vi "Compile Settings.vi"(8 "error in (no error)":errorcluster, 11 "Plugin in":refnum<class "Output Sequencer.lvclass">) -> (0 "error out":errorcluster, 3 "Plugin out":refnum<class "Output Sequencer.lvclass">)   [LabVIEW 2024, in "Output Sequencer.lvlib" / "Output Sequencer.lvclass"]
uses:
  Output Sequencer.lvclass
  Output Sequencer.lvclass/Output Sequencer.ctl
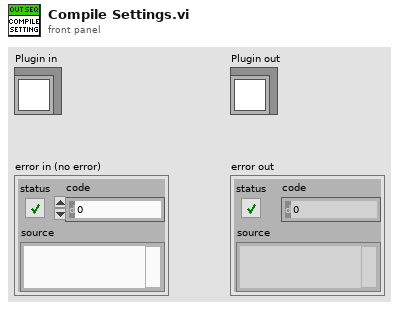
[diagram p1: front panel]
types:
  T1 = typedef "Output Sequencer.lvlib/Output Sequencer.lvclass/Expression Data.ctl" = cluster{"Empty?":bool, "Expression":refnum<class "mupExpr.lvclass">, "Variable Names":string[]}
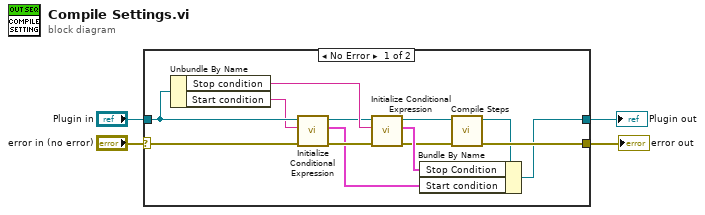
[diagram p0: block diagram]
diagram:
  n1 = case shown="No Error" "error in (no error)" {
    selector: "error in (no error)" -> [w5 w19]
    tunnel: [w17 w19] -> w4
    tunnel: [w16 w18] -> w3
    tunnel: "Plugin in" -> [w15 w18]
    frame No Error {
      n2 = Unbundle By Name(w15) -> ("Stop condition"=w13:string, "Start condition"=w14:string)
      n3 = call "Initialize Conditional Expression.vi"("error in (no error)"=w5, "Expression string"=w14, "Output Sequencer in"=w15) -> ("error out"=w11:errorcluster, "Expression Data"=w9:T1, "Output Sequencer out"=w12:refnum<class "Output Sequencer.lvclass">)  [unwired: 6 in]
      n4 = call "Initialize Conditional Expression.vi"("error in (no error)"=w11, "Expression string"=w13, "Output Sequencer in"=w12) -> ("error out"=w7:errorcluster, "Expression Data"=w10:T1, "Output Sequencer out"=w8:refnum<class "Output Sequencer.lvclass">)  [unwired: 6 in]
      n5 = call "Compile Steps.vi"("error in (no error)"=w7, "Plugin in"=w8) -> ("error out"=w17:errorcluster, "Plugin out"=w6:refnum<class "Output Sequencer.lvclass">)  [unwired: 8 in]
      n6 = Bundle By Name(cluster=w6, "Stop Condition"=w10, "Start condition"=w9) -> (w16:refnum<class "Output Sequencer.lvclass">)
    }
    frame Error {
    }
  }
  "error out" <- w4
  "Plugin out" <- w3
